vi "Lint VI Controls.vi"(8 "Error In":errorcluster, 11 "VI In":refnum<vi>) -> (0 "Error Out":errorcluster, 2 "Results":T1[](array[typedef]), 3 "VI Out":refnum<vi>)   [LabVIEW 2018, in "Scripts.lvlib"]
uses:
  Scripts.lvlib
  VI Control Lint Result.ctl
  <vilib>/Utility/traverseref.llb/TRef TravTarget.ctl
  <vilib>/Utility/traverseref.llb/VI Scripting - Traverse.lvlib
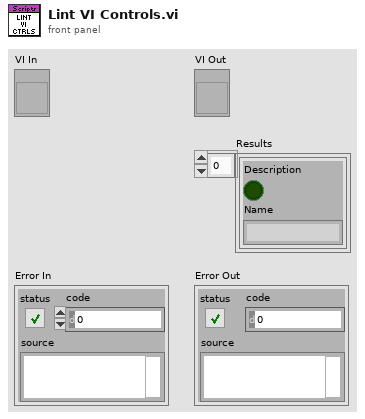
[diagram p1: front panel]
types:
  T1 = typedef "Scripts.lvlib/VI Control Lint Result.ctl" = cluster{"Description":bool, "Name":string}
  T2 = typedef "TRef TravTarget.ctl" = enum16{"FP", "BD", "Other"}
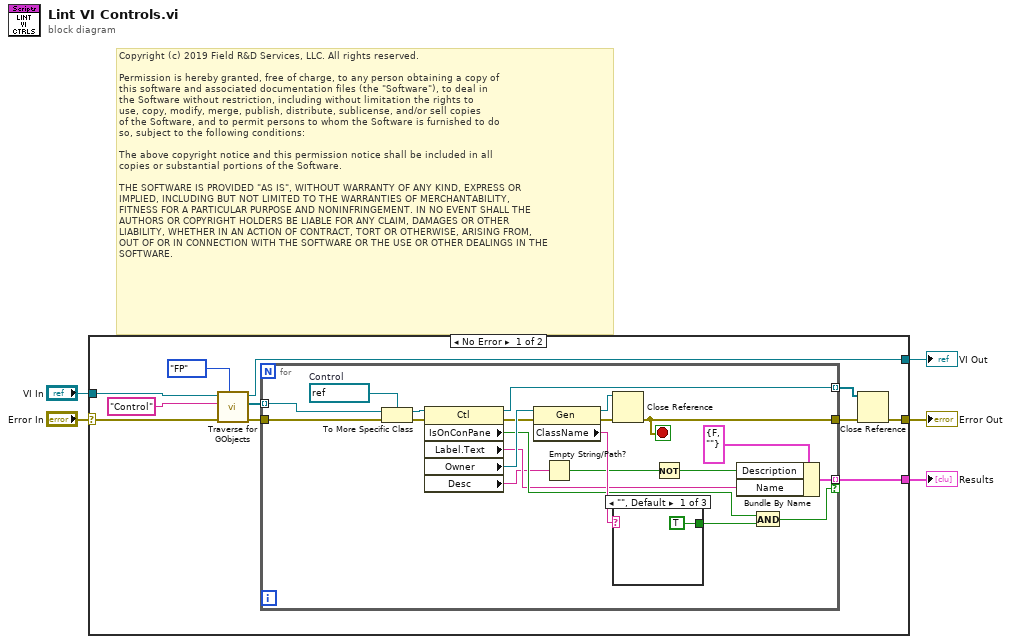
[diagram p0: block diagram]
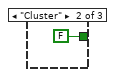
[diagram p2: hidden frame]
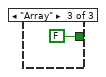
[diagram p3: hidden frame]
diagram:
  # "Copyright (c) 2019 Field R&D Services, LLC. All rights reserved.\n\nPermission is hereby granted, free of charge, to any person obtaining a copy of\nthis software and associated documentation files (the \"Software\"), to deal in\nthe Software without restriction, including without limitation the rights to\nuse, copy, modify, merge, publish, distribute, sublicense, and/or sell copies\nof the Software, and to permit persons to whom the Software is furnished to do\nso, subject to the following conditions:\n\nThe above copyright notice and this permission notice shall be included in all\ncopies or substantial portions of the Software.\n\nTHE SOFTWARE IS PROVIDED \"AS IS\", WITHOUT WARRANTY OF ANY KIND, EXPRESS OR\nIMPLIED, INCLUDING BUT NOT LIMITED TO THE WARRANTIES OF MERCHANTABILITY,\nFITNESS FOR A PARTICULAR PURPOSE AND NONINFRINGEMENT. IN NO EVENT SHALL THE\nAUTHORS OR COPYRIGHT HOLDERS BE LIABLE FOR ANY CLAIM, DAMAGES OR OTHER\nLIABILITY, WHETHER IN AN ACTION OF CONTRACT, TORT OR OTHERWISE, ARISING FROM,\nOUT OF OR IN CONNECTION WITH THE SOFTWARE OR THE USE OR OTHER DEALINGS IN THE\nSOFTWARE."
  n1 = case shown="No Error" "Error In" {
    selector: "Error In" -> [w10 w41]
    tunnel: "VI In" -> [w6 w42]
    tunnel: [w13 w42] -> w4
    tunnel: [w7 w41] -> w3
    tunnel: [w15 _] -> w2
    frame No Error {
      n2 = call <vilib>:"Traverse for GObjects.vi"("Traverse Target"=TRef_TravTarget."FP", "error in (no error)"=w10, "Class Name"="Control", "VI Refnum"=w6) -> ("error out"=w8:errorcluster, "References"=w9:refnum<vi>[], "dup VI Refnum"=w13:refnum<vi>)  [unwired: 4 in, 1 out]
      n3 = for {
        tunnel: [w37] -> w16 mode=indexing
        tunnel: [w36] -> w15 mode=indexing if=w25
        tunnel: [w21] -> w14
        tunnel: w9 -> [w34] mode=indexing
        tunnel: w8 -> [w30]
        stop <- w21 stop-if-true
        w32 = refnum<vi> refnum  # Control
        n4 = To More Specific Class(target class=w32, reference=w34, error in=w30) -> (specific class reference=w33:refnum<vi>, error out=w31:errorcluster)
        n5 = property class="Ctl"(reference=w33, error in=w31) -> (reference out=w37:refnum<vi>, error out=w24:errorcluster, "IsOnConPane"=w27:bool, "Label.Text"=w20:string, "Owner"=w29:refnum<vi>, "Desc"=w19:string)
        n6 = property class="Gen"(reference=w29, error in=w24) -> (reference out=w23:refnum<vi>, error out=w22:errorcluster, "ClassName"=w28:string)
        n7 = Empty String/Path?(string/path=w19) -> (empty?=w18:bool)
        n8 = Close Reference(reference=w23, error in (no error)=w22) -> (error out=w21:errorcluster)
        n9 = case shown="\"\", Default" w28 {
          tunnel: [TRUE FALSE FALSE] -> w26
          frame "", Default {
          }
          frame "Cluster" {
          }
          frame "Array" {
          }
        }
        n10 = Not(x=w18) -> (.not. x?=w17:bool)
        n11 = Bundle By Name(cluster=T1 {"Description"=FALSE, "Name"=""} ("VI Control Lint Result"), "Description"=w17, "Name"=w20) -> (w36:T1)
        n12 = And(x=w27, y=w26) -> (x .and. y?=w25:bool)
      }
      n13 = Close Reference(reference=w16, error in (no error)=w14) -> (error out=w7:errorcluster)
    }
    frame Error {
    }
  }
  "VI Out" <- w4
  "Error Out" <- w3
  "Results" <- w2
